vi "PAN_ObsFinishMngr.vi"(10 "nodeID":string, 11 "notifier":refnum<notifier>) -> ()   [LabVIEW 2016]
uses:
  PAN_ObsFinishStruct.ctl
panel:
  in  "Cluster":T1
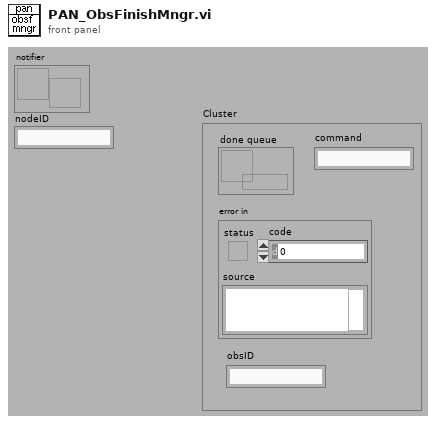
[diagram p1: front panel]
types:
  T1 = typedef "PAN_ObsFinishStruct.ctl" = cluster{"done queue":refnum<queue>, "error in":errorcluster, "obsID":string, "command":string}
  T2 = enum16{"add", "delete", "clean", "shutdown", "hold", "continue", "modify"}
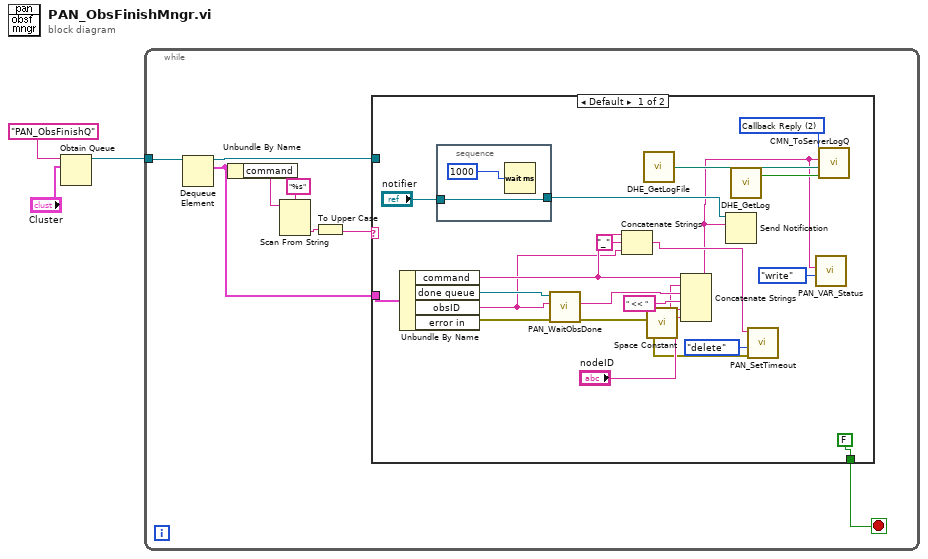
[diagram p0: block diagram]
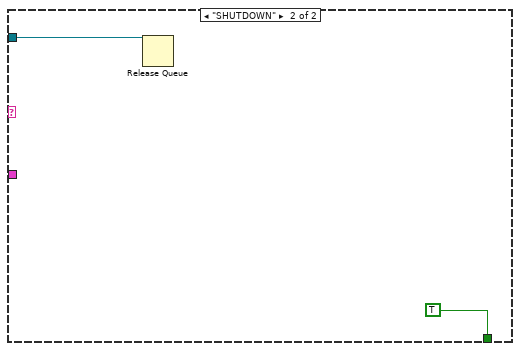
[diagram p2: hidden frame]
diagram:
  n1 = Obtain Queue(name (unnamed)="PAN_ObsFinishQ", element data type="Cluster") -> (queue out=w2:refnum<queue>)  [unwired: 3 in, 2 out]
  n2 = while {
    tunnel: w2 -> [w11]
    stop <- w5 stop-if-true
    n3 = Dequeue Element(queue=w11) -> (queue out=w6:refnum<queue>, element=w4:T1)  [unwired: 1 in, 3 out]
    n4 = Unbundle By Name(w4) -> ("command"=w10:string)
    n5 = Scan From String(format string="%s", input string=w10) -> (output 1=w8:string)  [unwired: 2 in, 4 out]
    n6 = To Upper Case(1:w8) -> (0:w7:string)
    n7 = case shown="Default" w7 {
      tunnel: w6 -> [_ w36]
      tunnel: [FALSE TRUE] -> w5
      tunnel: w4 -> [w31 _]
      frame Default {
        w20 = u16 2 items=["command", "imediateReply", "Callback Reply", "Information"] ("type")
        n8 = Unbundle By Name(w31) -> ("command"=w17:string, "done queue"=w30:refnum<queue>, "obsID"=w14:string, "error in"=w29:errorcluster)
        n9 = stacked-sequence {
          tunnel: [w33] -> w18
          tunnel: "notifier" -> [w33]
          frame #0 {
            n10 = Wait (ms)(milliseconds to wait=u32 1000) -> ()  [unwired: 1 out]
          }
        }
        n11 = call "PAN_WaitObsDone.vi"("error in"=w29, "obsID"=w14, "done queue"=w30) -> ("error out"=w24:errorcluster, "response"=w27:string)  [unwired: 7 out]
        n12 = Concatenate Strings(w17, "_" ("string"), w14) -> (w15:string)
        n13 = call "DHE_GetLogFile.vi"() -> ("DHE_LogFile"=w22:path)  [unwired: 9 out]
        n14 = call <vilib>:"Space Constant.vi"() -> ("String"=w26:string)
        n15 = Concatenate Strings(w17, w26, w27, " << " ("string"), "nodeID", w26) -> (w13:string)
        n16 = Send Notification(notification=w13, notifier=w18) -> ()  [unwired: 1 in, 2 out]
        n17 = call "DHE_GetLog.vi"() -> ("DHE_log"=w21:bool)  [unwired: 9 out]
        n18 = call "PAN_SetTimeout.vi"("error in (no error)"=w24, "action"=T2."delete", "Command"=w15) -> ()  [unwired: 1 in, 8 out]
        n19 = call "PAN_VAR_Status.vi"("action"=enum16{"read", "write", "set_ref"}."write", "status in"=w13) -> ()  [unwired: 2 in, 8 out]
        n20 = call "CMN_ToServerLogQ.vi"("Log"=w21, "file"=w22, "string"=w13, "type"=w20) -> ()  [unwired: 2 in, 5 out]
      }
      frame "SHUTDOWN" {
        n21 = Release Queue(queue=w36) -> ()  [unwired: 1 in, 4 out]
      }
    }
  }
